vi "Remove Named Gate Prefix.vi"(1 "name in":string) -> (0 "name out":string)   [LabVIEW 2015, in "Gates.lvlib"]
doc: "Searches and removes \"CustomSemaphore.Gate.\" from the <b>name in</b>."
uses:
  Gates.lvlib
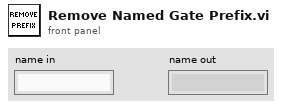
[diagram p1: front panel]
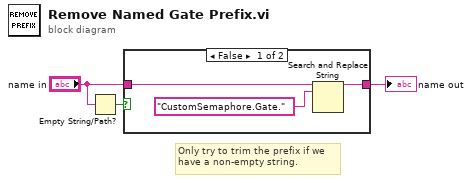
[diagram p0: block diagram]
diagram:
  # "Only try to trim the prefix if we\nhave a non-empty string."
  n1 = Empty String/Path?(string/path="name in") -> (empty?=w3:bool)
  n2 = case shown="False" w3 {
    tunnel: "name in" -> [w6 w7]
    tunnel: [w4 w7] -> w1
    frame False {
      n3 = Search and Replace String(input string=w6, search string="CustomSemaphore.Gate." ("string")) -> (result string=w4:string)  [unwired: 1 in, 8 out]
    }
    frame True {
    }
  }
  "name out" <- w1
